vi "Configuration.vi"(7 "Get/Set":enum16{"Get menu", "Update menu"}(ring), 8 "Error In":errorcluster, 10 "Path":path, 11 "Menus":T1(array[cluster])) -> (0 "Error Out":errorcluster, 3 "Menus out":T1(array[cluster]))   [LabVIEW 2019]
uses:
  <vilib>/Utility/config.llb/Read Key (String).vi
  <vilib>/Utility/config.llb/Read Key (U32).vi
  <vilib>/Utility/config.llb/Read Key (Boolean).vi
  <vilib>/Utility/config.llb/Read Key (I32).vi
  <vilib>/Utility/config.llb/Write Key (I32).vi
  <vilib>/Utility/config.llb/Write Key (String).vi
  <vilib>/Utility/config.llb/Write Key (U32).vi
  <vilib>/Utility/config.llb/Write Key (Boolean).vi
  <vilib>/Utility/config.llb/NI_LVConfig.lvlib
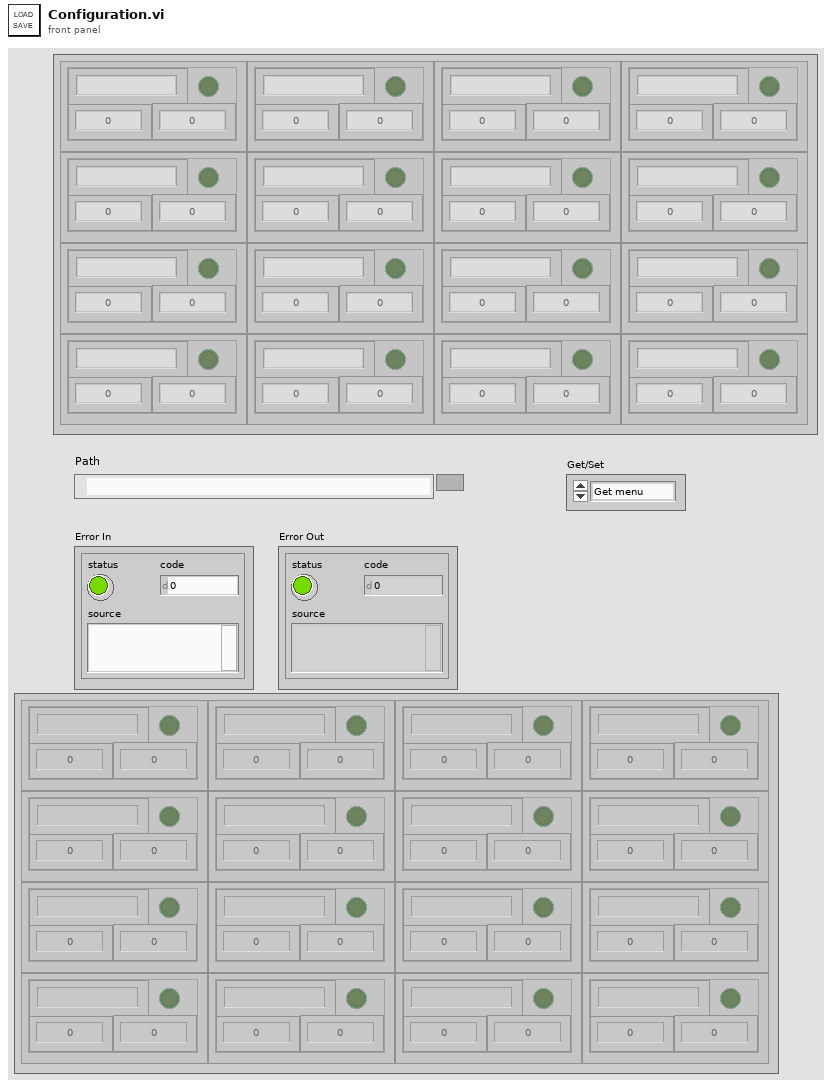
[diagram p1: front panel]
types:
  T1 = cluster{"Price":u32, "Name":string, "Left":u32, "Available":bool}[][]
  T2 = typedef "NI_LVConfig.lvlib/Config Data RefNum.ctl" = refnum<k1>
  T3 = cluster{"Price":u32, "Name":string, "Left":u32, "Available":bool}
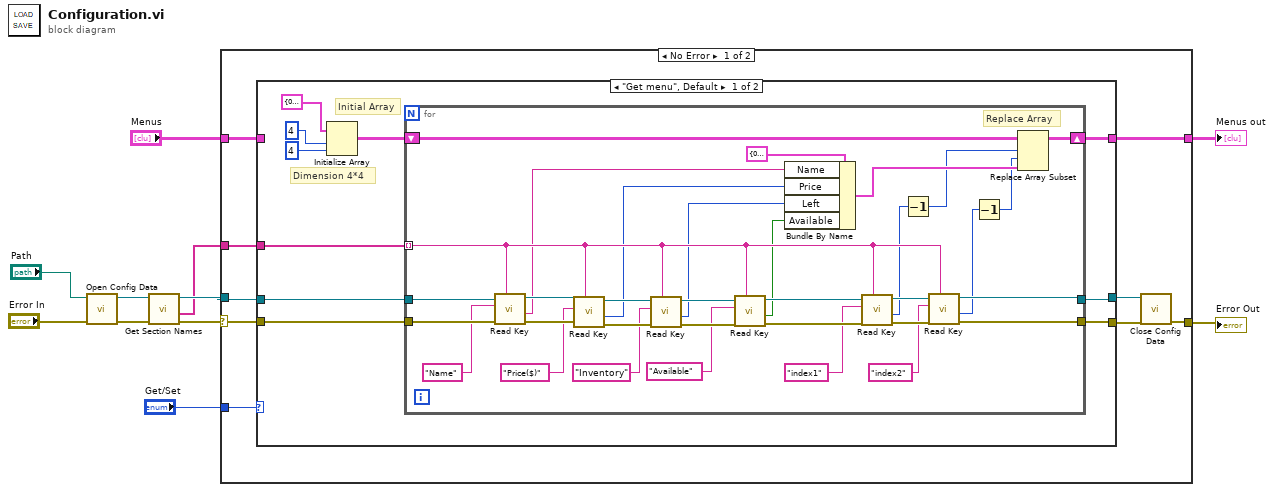
[diagram p0: block diagram]
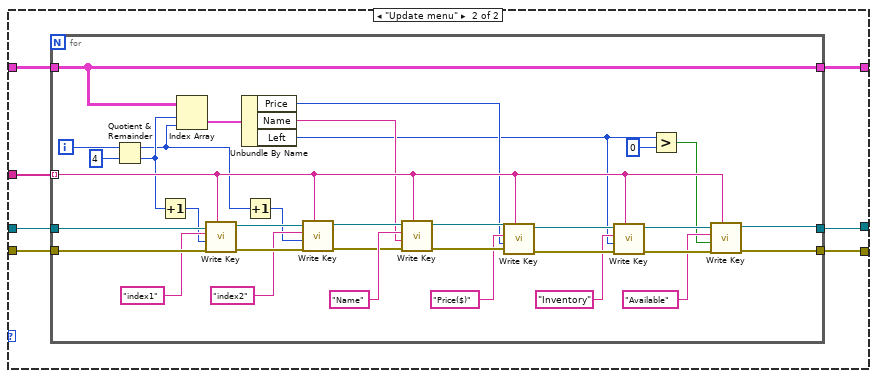
[diagram p2: hidden frame]
diagram:
  n1 = call <vilib>:"Open Config Data.vi"("error in (no error)"="Error In", "configuration file path"="Path") -> ("error out"=w9:errorcluster, "refnum"=w8:T2)  [unwired: 7 in, 1 out]
  n2 = call <vilib>:"Get Section Names.vi"("error in (no error)"=w9, "refnum"=w8) -> ("error out"=w7:errorcluster, "section names"=w5:string[], "refnum out"=w6:T2)  [unwired: 7 in]
  n3 = case shown="No Error" w7 {
    selector: w7 -> [w20 w105]
    tunnel: [w12 w105] -> w3
    tunnel: "Menus" -> [w19 w106]
    tunnel: "Get/Set" -> [w18 _]
    tunnel: [w17 w106] -> w2
    tunnel: w6 -> [w16 _]
    tunnel: w5 -> [w15 _]
    frame No Error {
      n4 = case shown="\"Get menu\", Default" w18 {
        tunnel: w20 -> [w30 w70]
        tunnel: [w27 w68] -> w14
        tunnel: w16 -> [w29 w69]
        tunnel: w15 -> [w28 w66]
        tunnel: [w26 w67] -> w13
        tunnel: [w21 w64] -> w17
        tunnel: w19 -> [_ w65]
        frame "Get menu", Default {
          # "Initial Array"
          # "Dimension 4*4"
          n5 = Initialize Array(T3 {"Price"=0, "Name"="", "Left"=0, "Available"=FALSE} ("Items"), 4 ("dimension size"), 4 ("dimension size")) -> (w22:T1)
          n6 = for {
            tunnel: w30 -> [w63]
            tunnel: w28 -> [w43] mode=indexing
            tunnel: [w45] -> w27
            shift-right: [w35] -> w21
            shift-left: w22 -> [w37]
            tunnel: w29 -> [w62]
            tunnel: [w44] -> w26
            # "Replace Array"
            n7 = call-poly <vilib>:"Read Key.vi"("section"=w43, "error in (no error)"=w63, "key"="Name", "refnum"=w62) -> ("error out"=w60:errorcluster, "value"=w42:string, "refnum out"=w59:T2)  [unwired: 4 in, 1 out]
            n8 = call-poly <vilib>:"Read Key.vi"("section"=w43, "error in (no error)"=w60, "key"="Price($)", "refnum"=w59) -> ("error out"=w57:errorcluster, "value"=w41:u32, "refnum out"=w56:T2)  [unwired: 4 in, 1 out]
            n9 = call-poly <vilib>:"Read Key.vi"("section"=w43, "error in (no error)"=w57, "key"="Inventory", "refnum"=w56) -> ("error out"=w54:errorcluster, "value"=w40:u32, "refnum out"=w53:T2)  [unwired: 4 in, 1 out]
            n10 = call-poly <vilib>:"Read Key.vi"("section"=w43, "error in (no error)"=w54, "key"="Available", "refnum"=w53) -> ("error out"=w50:errorcluster, "value"=w38:bool, "refnum out"=w51:T2)  [unwired: 4 in, 1 out]
            n11 = Bundle By Name(cluster=T3 {"Price"=0, "Name"="", "Left"=0, "Available"=FALSE} ("Items"), "Name"=w42, "Price"=w41, "Left"=w40, "Available"=w38) -> (w36:T3)
            n12 = call-poly <vilib>:"Read Key.vi"("section"=w43, "error in (no error)"=w50, "key"="index1", "refnum"=w51) -> ("error out"=w48:errorcluster, "value"=w34:i32, "refnum out"=w47:T2)  [unwired: 4 in, 1 out]
            n13 = Decrement(x=w34) -> (x-1=w32:i32)
            n14 = call-poly <vilib>:"Read Key.vi"("section"=w43, "error in (no error)"=w48, "key"="index2", "refnum"=w47) -> ("error out"=w45:errorcluster, "value"=w33:i32, "refnum out"=w44:T2)  [unwired: 4 in, 1 out]
            n15 = Decrement(x=w33) -> (x-1=w31:i32)
            n16 = Replace Array Subset(array=w37, new element=w36, index (row)=w32, index (col)=w31) -> (w35:T1)
          }
        }
        frame "Update menu" {
          n17 = for {
            tunnel: w70 -> [w103]
            tunnel: w66 -> [w100] mode=indexing
            tunnel: [w101] -> w68
            tunnel: w65 -> [w81]
            tunnel: [w81] -> w64
            tunnel: w69 -> [w104]
            tunnel: [w102] -> w67
            i -> [w76]
            n18 = Quotient & Remainder(x=w76, y=4) -> (x-y*floor(x/y)=w74:i32, floor(x/y)=w75:i32)
            n19 = Increment(x=w75) -> (x+1=w78:i32)
            n20 = Index Array(array=w81, index (row)=w75, index (col)=w74) -> (element=w80:T3)
            n21 = call-poly <vilib>:"Write Key.vi"("section"=w100, "error in (no error)"=w103, "value"=w78, "key"="index1", "refnum"=w104) -> ("error out"=w88:errorcluster, "refnum out"=w87:T2)  [unwired: 4 in, 1 out]
            n22 = Unbundle By Name(w80) -> ("Price"=w82:u32, "Name"=w83:string, "Left"=w73:u32)
            n23 = Increment(x=w74) -> (x+1=w77:i32)
            n24 = call-poly <vilib>:"Write Key.vi"("section"=w100, "error in (no error)"=w88, "value"=w77, "key"="index2", "refnum"=w87) -> ("error out"=w85:errorcluster, "refnum out"=w84:T2)  [unwired: 4 in, 1 out]
            n25 = call-poly <vilib>:"Write Key.vi"("section"=w100, "error in (no error)"=w85, "value"=w83, "key"="Name", "refnum"=w84) -> ("error out"=w98:errorcluster, "refnum out"=w97:T2)  [unwired: 4 in, 1 out]
            n26 = call-poly <vilib>:"Write Key.vi"("section"=w100, "error in (no error)"=w98, "value"=w82, "key"="Price($)", "refnum"=w97) -> ("error out"=w95:errorcluster, "refnum out"=w94:T2)  [unwired: 4 in, 1 out]
            n27 = call-poly <vilib>:"Write Key.vi"("section"=w100, "error in (no error)"=w95, "value"=w73, "key"="Inventory", "refnum"=w94) -> ("error out"=w92:errorcluster, "refnum out"=w91:T2)  [unwired: 4 in, 1 out]
            n28 = Greater?(x=w73, y=u32 0) -> (0:w71:bool)
            n29 = call-poly <vilib>:"Write Key.vi"("section"=w100, "error in (no error)"=w92, "value"=w71, "key"="Available", "refnum"=w91) -> ("error out"=w101:errorcluster, "refnum out"=w102:T2)  [unwired: 4 in, 1 out]
          }
        }
      }
      n30 = call <vilib>:"Close Config Data.vi"("error in (no error)"=w14, "refnum"=w13) -> ("error out"=w12:errorcluster)  [unwired: 8 in, 1 out]
    }
    frame Error {
    }
  }
  "Error Out" <- w3
  "Menus out" <- w2
